vi "Before Dig.vi"(8 "Error In":errorcluster, 11 "VI In":refnum<vi>) -> (0 "Error Out":errorcluster, 1 "Graves Count":i32, 2 "Selection List":refnum<vi>[](array[refnum]), 3 "VI Out":refnum<vi>)   [LabVIEW 2018, in "Tests.lvlib" / "Toolkit.lvlib" / "Integration.lvlib"]
uses:
  Integration.lvlib
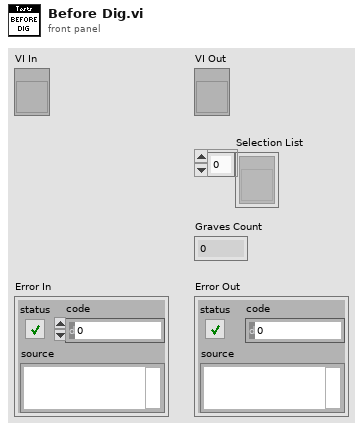
[diagram p1: front panel]
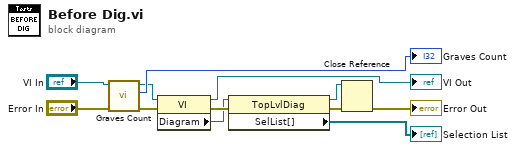
[diagram p0: block diagram]
diagram:
  n1 = call "Graves Count.vi"("Error In"="Error In", "Test Target In"="VI In") -> ("Error Out"=w6:errorcluster, "Graves Count"=→"Graves Count":i32, "Test Target Out"=w5:refnum<vi>)  [unwired: 7 in]
  n2 = property class="VI"(reference=w5, error in=w6) -> (reference out=→"VI Out":refnum<vi>, error out=w2:errorcluster, "Diagram"=w1:refnum<vi>)
  n3 = property class="TopLvlDiag"(reference=w1, error in=w2) -> (reference out=w4:refnum<vi>, error out=w3:errorcluster, "SelList[]"=→"Selection List":refnum<vi>[])
  n4 = Close Reference(reference=w4, error in (no error)=w3) -> (error out=→"Error Out":errorcluster)
